vi "SP Perform Filter Attenuation Limit Testing.vi"(6 "Limit Results In":T3={"Limit #"=0, "Parameter"={"Stimulus Port"=1, "Response Port"=0}, "Bandwidth Pass?"={"Pass?"=FALSE, "Bandwidth"=0.0, "Limit"=0.0, "Units"=enum."Hz"}, "Ripple Pass?"={"Pass?"=FALSE, "Ripple"=0.0, "Limit"=0.0, "Format"=enum."Log Mag"}, "Attenuation Results"=[], "Skirt Results"=[], "Pass?"=FALSE} {"Parameter"."Stimulus Port" min=1 step=1; "Parameter"."Response Port" min=1 step=1}, 8 "error in (no error)":errorcluster, 10 "Data":T11={"F0"=500.0, "dF"=1.0, "Formatted Values"=[-6.0, -6.0, -6.0, -6.0, -6.0, -6.0, -5.0, -4.0, -3.0, -2.0, -1.0017226002993769, -0.8636286738753696, -1.012432061728755, -0.8135188671805874, -1.084383696215112, -1.192695586219516, -0.8228939725524264, -1.1588169801015764, -1.0069715761898415, -0.8118111488159718, -0.9516999033989667, -1.0842662636672022, -1.0261931083967077, -0.816874162233468, -0.8335770068326294, -1.1794529347576463, -1.1032959879886735, -1.197742447623333, -0.9631229100196212, -0.9908453124177325, -0.9835470980893588, -1.10217991844936, -0.8956607286257672, -0.8794782872077156, -0.9013683651609963, -1.0772188731817596, -0.992723355191172, -0.9536275499498994, -0.9874327685983141, -0.921963653527827, -0.8848787728556787, -1.1874980208218, -0.996957511881206, -0.9972503730309241, -0.8866139538542095, -1.07344181331393, -0.881559772443858, -1.0112449407130875, -0.9865384477979471, -0.9901446738263366, -1.1718630063784758, -0.9951725256878827, -0.931778781153855, -0.9846289731021831, -0.851763264124267, -0.9086965469391421, -0.8349429101974368, -0.8383742350256687, -1.106571816484691, -0.9554005266395742, -0.9376822403043366, -1.131287512516927, -1.0382288806403288, -0.917054052988136, -0.9489467877812984, -0.9264227759143271, -1.0918690925892351, -1.1668737446636852, -1.0021735712381068, -1.1541225361979714, -1.1931131329605709, -0.8730502330378824, -0.850411285659811, -1.137775166801135, -1.1870586525662095, -1.0926571181161528, -1.118993526927924, -1.1211410787283602, -0.8920697041785735, -0.888430731015914, -1.0656600076605476, -1.1666787859795846, -1.0713340188424678, -0.8625910088884297, -1.1434360227216422, -0.9217710376784376, -1.1218396445954617, -0.9558195687190933, -1.1773692443654946, -1.0827782751424972, -1.1567791336122029, -0.8684407402614696, -0.8177845157195978, -0.9040657051180614, -0.9313557288389804, -1.0236831450620423, -1.050426714979035, -0.8344777069605718, -0.8274082929927138, -1.1990080831766776, -1.0947798998491134, -1.1963114865246718, -1.0016247375583676, -1.0877110100652403, -1.1556028882288836, -1.1918380581525247, -0.9751292214691399, -0.8884133044813358, -1.0347444321214612, -0.9445125246491541, -2.0, -3.0, -4.0, -5.0, -6.0, -6.0, -6.0, -6.0, -6.0, -6.0]}, 11 "Filter Limit":T12={"Limit #"=1, "Parameter"={"Stimulus Port"=1, "Response Port"=2}, "Format"=enum."Lin Mag", "Filter Type"=enum."Bandpass", "Passband"={"Start/Center"=510.0, "Stop/Span"=610.0, "Units"=enum."MHz", "Freq Format"=enum."Start/Stop", "Bandwidth Attn"=3.0, "Passband Limit"=FALSE}, "Ripple"={"Ripple Limit"=TRUE, "Window On"=FALSE, "Ripple"=0.1, "Window"=10.0, "Units"=enum."MHz"}, "Attenuation Points"=[{"Attenuation"=3.0, "Type"=enum."Center", "Lower"=10.0, "Upper"=10.0, "Units"=enum."MHz"}], "Skirt Points"=[]} {"Parameter"."Stimulus Port" min=1 step=1; "Parameter"."Response Port" min=1 step=1; "Passband"."Bandwidth Attn" format="%.3g"; "Passband"."Stop/Span" format="%.3g"; "Passband"."Start/Center" format="%.3g"}) -> (0 "error out":errorcluster, 1 "Failures":cluster{"x values":dbl[], "y values":dbl[]}[](array[cluster]), 2 "Results":T2(array[cluster]), 3 "Pass?":bool=TRUE, 4 "Limit Results Out":T3={"Limit #"=0, "Parameter"={"Stimulus Port"=1, "Response Port"=0}, "Bandwidth Pass?"={"Pass?"=FALSE, "Bandwidth"=0.0, "Limit"=0.0, "Units"=enum."Hz"}, "Ripple Pass?"={"Pass?"=FALSE, "Ripple"=0.0, "Limit"=0.0, "Format"=enum."Log Mag"}, "Attenuation Results"=[], "Skirt Results"=[], "Pass?"=FALSE} {"Parameter"."Stimulus Port" min=1 step=1; "Parameter"."Response Port" min=1 step=1}, 5 "Lower Limits":cluster{"x values":dbl[], "y values":dbl[]}[](array[cluster])=[{"x values"=[550.0, 550.0], "y values"=[-inf, inf]}], 7 "Upper Limits":cluster{"x values":dbl[], "y values":dbl[]}[](array[cluster])=[{"x values"=[570.0, 570.0], "y values"=[-inf, inf]}])   [LabVIEW 2011]
uses:
  TypeDefs/SP Filter.ctl
  TypeDefs/SP Parameter.ctl
  TypeDefs/SP Format.ctl
  TypeDefs/SP Filter Type.ctl
  TypeDefs/SP Filter Passband.ctl
  TypeDefs/SP Frequency Units.ctl
  TypeDefs/SP Frequency Format.ctl
  TypeDefs/SP Filter Ripple.ctl
  TypeDefs/SP Attenuation Point.ctl
  TypeDefs/SP Attenuation Type.ctl
  TypeDefs/SP Skirt Rejection Point.ctl
  TypeDefs/SP Relative Loss.ctl
  TypeDefs/SP Limit Results.ctl
  TypeDefs/SP Bandwidth Limit Results.ctl
  TypeDefs/SP Ripple Limit Results.ctl
  TypeDefs/SP Attenuation Limit Results.ctl
  TypeDefs/SP Skirt Limit Results.ctl
panel:
  out "Plot Output":cluster{"x values":dbl[], "y values":dbl[]}[](graph)=[{"x values"=[], "y values"=[]}, {"x values"=[570.0, 570.0], "y values"=[-inf, inf]}, {"x values"=[550.0, 550.0], "y values"=[-inf, inf]}, {"x values"=[500.0, 501.0, 502.0, 503.0, 504.0, 505.0, 506.0, 507.0, 508.0, 509.0, 510.0, 511.0, 512.0, 513.0, 514.0, 515.0, 516.0, 517.0, 518.0, 519.0, 520.0, 521.0, 522.0, 523.0, 524.0, 525.0, 526.0, 527.0, 528.0, 529.0, 530.0, 531.0, 532.0, 533.0, 534.0, 535.0, 536.0, 537.0, 538.0, 539.0, 540.0, 541.0, 542.0, 543.0, 544.0, 545.0, 546.0, 547.0, 548.0, 549.0, 550.0, 551.0, 552.0, 553.0, 554.0, 555.0, 556.0, 557.0, 558.0, 559.0, 560.0, 561.0, 562.0, 563.0, 564.0, 565.0, 566.0, 567.0, 568.0, 569.0, 570.0, 571.0, 572.0, 573.0, 574.0, 575.0, 576.0, 577.0, 578.0, 579.0, 580.0, 581.0, 582.0, 583.0, 584.0, 585.0, 586.0, 587.0, 588.0, 589.0, 590.0, 591.0, 592.0, 593.0, 594.0, 595.0, 596.0, 597.0, 598.0, 599.0, 600.0, 601.0, 602.0, 603.0, 604.0, 605.0, 606.0, 607.0, 608.0, 609.0, 610.0, 611.0, 612.0, 613.0, 614.0, 615.0, 616.0, 617.0, 618.0, 619.0], "y values"=[-6.0, -6.0, -6.0, -6.0, -6.0, -6.0, -5.0, -4.0, -3.0, -2.0, -1.0017226002993769, -0.8636286738753696, -1.012432061728755, -0.8135188671805874, -1.084383696215112, -1.192695586219516, -0.8228939725524264, -1.1588169801015764, -1.0069715761898415, -0.8118111488159718, -0.9516999033989667, -1.0842662636672022, -1.0261931083967077, -0.816874162233468, -0.8335770068326294, -1.1794529347576463, -1.1032959879886735, -1.197742447623333, -0.9631229100196212, -0.9908453124177325, -0.9835470980893588, -1.10217991844936, -0.8956607286257672, -0.8794782872077156, -0.9013683651609963, -1.0772188731817596, -0.992723355191172, -0.9536275499498994, -0.9874327685983141, -0.921963653527827, -0.8848787728556787, -1.1874980208218, -0.996957511881206, -0.9972503730309241, -0.8866139538542095, -1.07344181331393, -0.881559772443858, -1.0112449407130875, -0.9865384477979471, -0.9901446738263366, -1.1718630063784758, -0.9951725256878827, -0.931778781153855, -0.9846289731021831, -0.851763264124267, -0.9086965469391421, -0.8349429101974368, -0.8383742350256687, -1.106571816484691, -0.9554005266395742, -0.9376822403043366, -1.131287512516927, -1.0382288806403288, -0.917054052988136, -0.9489467877812984, -0.9264227759143271, -1.0918690925892351, -1.1668737446636852, -1.0021735712381068, -1.1541225361979714, -1.1931131329605709, -0.8730502330378824, -0.850411285659811, -1.137775166801135, -1.1870586525662095, -1.0926571181161528, -1.118993526927924, -1.1211410787283602, -0.8920697041785735, -0.888430731015914, -1.0656600076605476, -1.1666787859795846, -1.0713340188424678, -0.8625910088884297, -1.1434360227216422, -0.9217710376784376, -1.1218396445954617, -0.9558195687190933, -1.1773692443654946, -1.0827782751424972, -1.1567791336122029, -0.8684407402614696, -0.8177845157195978, -0.9040657051180614, -0.9313557288389804, -1.0236831450620423, -1.050426714979035, -0.8344777069605718, -0.8274082929927138, -1.1990080831766776, -1.0947798998491134, -1.1963114865246718, -1.0016247375583676, -1.0877110100652403, -1.1556028882288836, -1.1918380581525247, -0.9751292214691399, -0.8884133044813358, -1.0347444321214612, -0.9445125246491541, -2.0, -3.0, -4.0, -5.0, -6.0, -6.0, -6.0, -6.0, -6.0, -6.0]}]
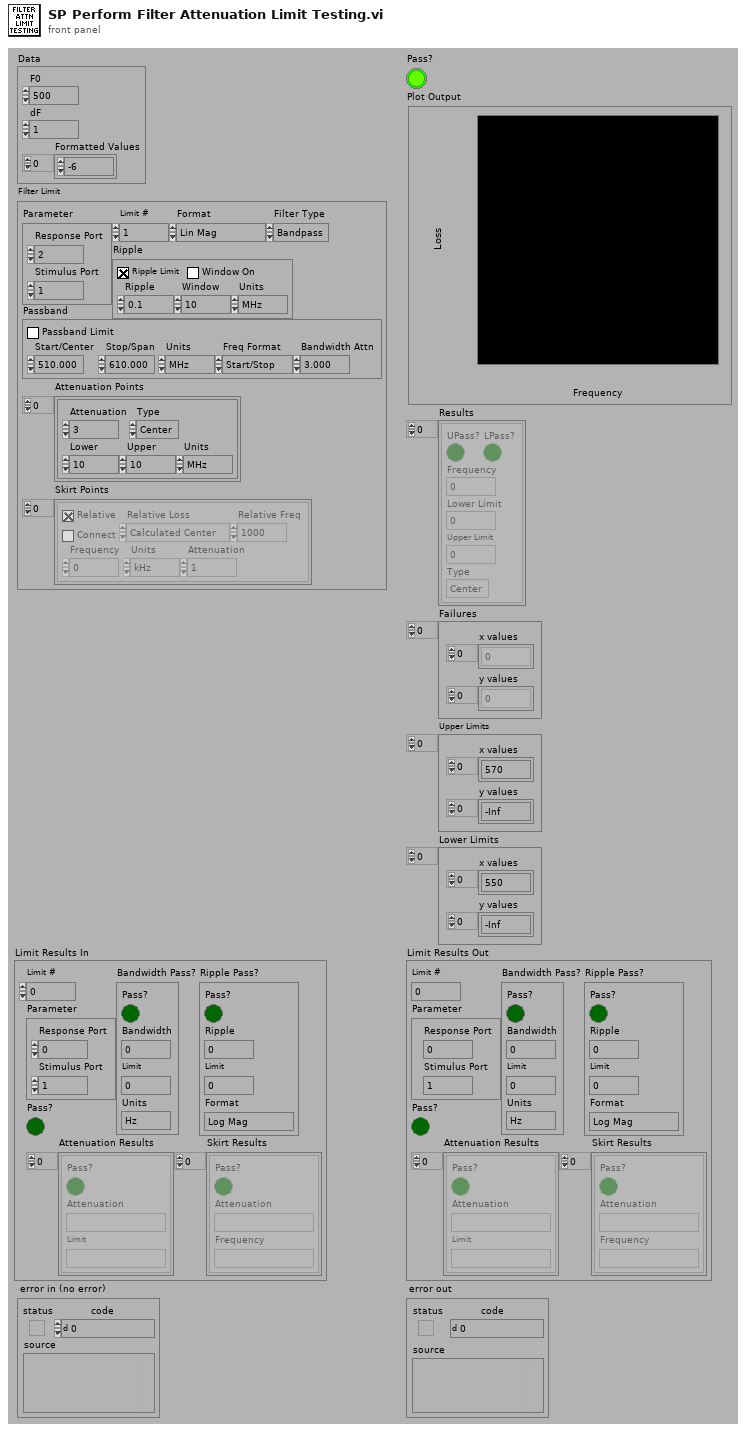
[diagram p1: front panel]
types:
  T1 = typedef "SP Attenuation Type.ctl" = enum16{"Center", "Lower", "Upper"}
  T2 = cluster{"UPass?":bool, "LPass?":bool, "Frequency":dbl, "Lower Limit":dbl, "Upper Limit":dbl, "Type":T1}[]
  T3 = typedef "SP Limit Results.ctl" = cluster{"Limit #":i8, "Parameter":T4, "Bandwidth Pass?":T5, "Ripple Pass?":T7, "Attenuation Results":T9[], "Skirt Results":T10[], "Pass?":bool}
  T4 = typedef "SP Parameter.ctl" = cluster{"Stimulus Port":i8, "Response Port":i8}
  T5 = typedef "SP Bandwidth Limit Results.ctl" = cluster{"Pass?":bool, "Bandwidth":dbl, "Limit":dbl, "Units":T6}
  T6 = typedef "SP Frequency Units.ctl" = enum16{"Hz", "kHz", "MHz", "GHz", "Points"}
  T7 = typedef "SP Ripple Limit Results.ctl" = cluster{"Pass?":bool, "Ripple":dbl, "Limit":dbl, "Format":T8}
  T8 = typedef "SP Format.ctl" = enum16{"Log Mag", "Lin Mag", "SWR", "Phase", "Expanded Phase", "Delay", "Insertion Loss", "Isolation", "Return Loss"}
  T9 = typedef "SP Attenuation Limit Results.ctl" = cluster{"Pass?":bool, "Attenuation":string, "Limit":string}
  T10 = typedef "SP Skirt Limit Results.ctl" = cluster{"Pass?":bool, "Attenuation":string, "Frequency":string}
  T11 = cluster{"F0":dbl, "dF":dbl, "Formatted Values":dbl[]}
  T12 = typedef "SP Filter.ctl" = cluster{"Limit #":i8, "Parameter":T4, "Format":T8, "Filter Type":T13, "Passband":T14, "Ripple":T16, "Attenuation Points":T17[], "Skirt Points":T18[]}
  T13 = typedef "SP Filter Type.ctl" = enum16{"Lowpass", "Highpass", "Bandpass", "Bandstop"}
  T14 = typedef "SP Filter Passband.ctl" = cluster{"Start/Center":dbl, "Stop/Span":dbl, "Units":T6, "Freq Format":T15, "Bandwidth Attn":dbl, "Passband Limit":bool}
  T15 = typedef "SP Frequency Format.ctl" = enum16{"Start/Stop", "Center/Span"}
  T16 = typedef "SP Filter Ripple.ctl" = cluster{"Ripple Limit":bool, "Window On":bool, "Ripple":dbl, "Window":dbl, "Units":T6}
  T17 = typedef "SP Attenuation Point.ctl" = cluster{"Attenuation":dbl, "Type":T1, "Lower":dbl, "Upper":dbl, "Units":T6}
  T18 = typedef "SP Skirt Rejection Point.ctl" = cluster{"Relative":bool, "Connect":bool, "Frequency":dbl, "Units":T6, "Attenuation":dbl, "Relative Loss":T19, "Relative Freq":dbl}
  T19 = typedef "SP Relative Loss.ctl" = enum16{"Calculated Center", "Passband Minimum", "Passband Maximum", "Passband Average", "Frequency"}
  T20 = cluster{bool, bool, "Interpolated X Value":dbl, dbl, dbl, "Type":T1}
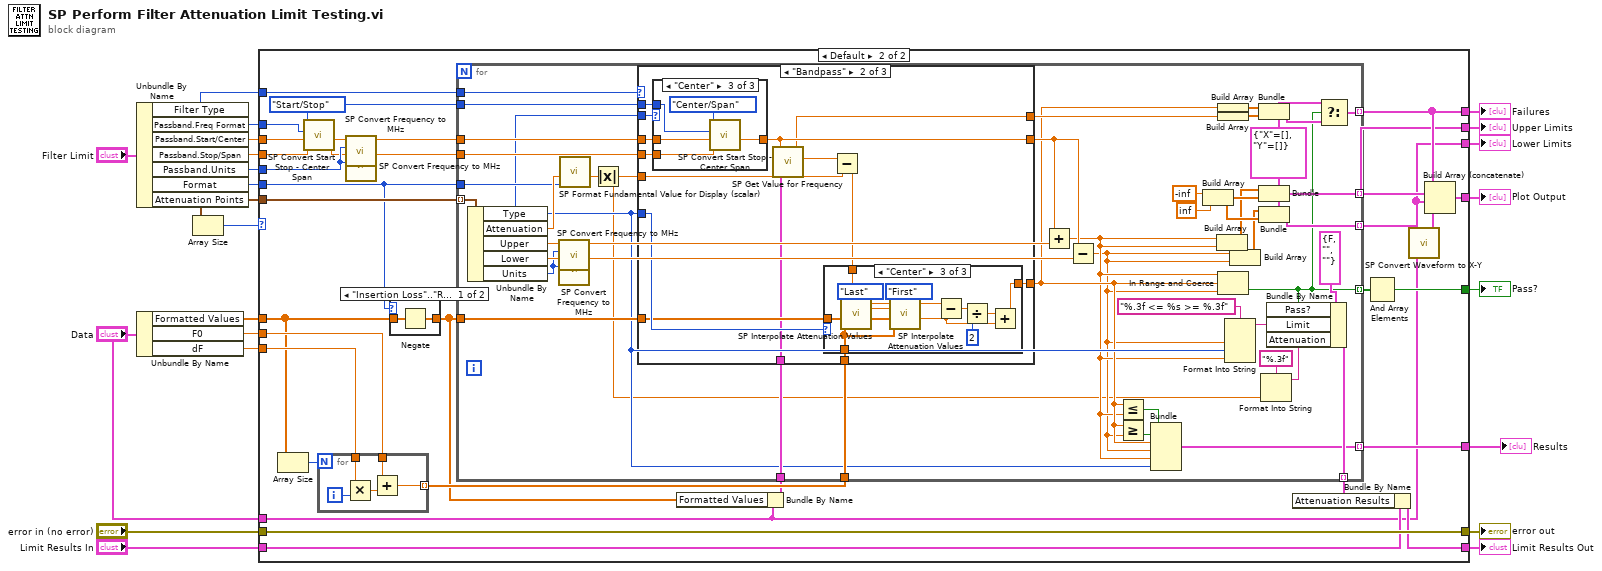
[diagram p0: block diagram]
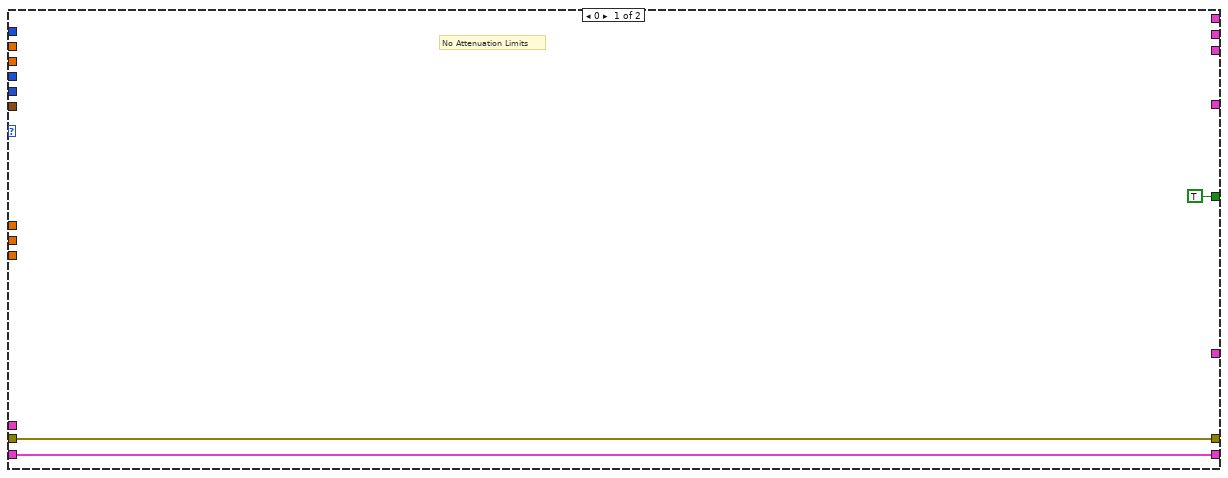
[diagram p2: hidden frame]
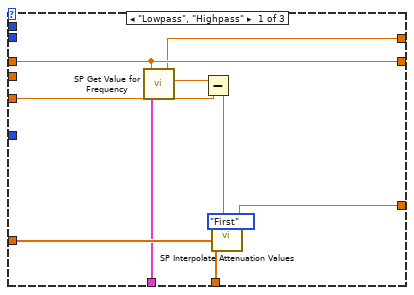
[diagram p4: hidden frame]
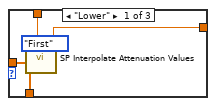
[diagram p5: hidden frame]
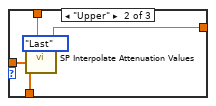
[diagram p6: hidden frame]
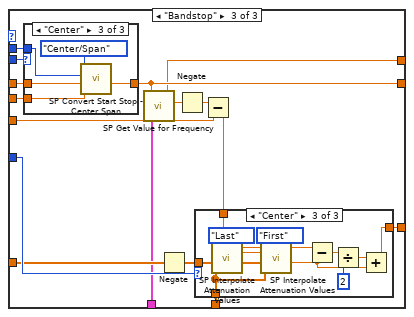
[diagram p9: hidden frame]
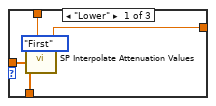
[diagram p10: hidden frame]
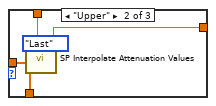
[diagram p11: hidden frame]
diagram:
  n1 = Unbundle By Name("Filter Limit") -> ("Filter Type"=w14:T13, "Passband.Freq Format"=w13:T15, "Passband.Start/Center"=w22:dbl, "Passband.Stop/Span"=w21:dbl, "Passband.Units"=w20:T6, "Format"=w11:T8, "Attenuation Points"=w12:T17[])
  n2 = Unbundle By Name("Data") -> ("Formatted Values"=w19:dbl[], "F0"=w8:dbl, "dF"=w7:dbl)
  n3 = Array Size(array=w12) -> (size(s)=w9:i32)
  n4 = case shown="Default" w9 {
    tunnel: w14 -> [_ w49]
    tunnel: w22 -> [_ w55]
    tunnel: w21 -> [_ w52]
    tunnel: w20 -> [_ w58]
    tunnel: w19 -> [_ w31]
    tunnel: w12 -> [_ w56]
    tunnel: "Data" -> [_ w29]
    tunnel: [TRUE w46] -> w17
    tunnel: "error in (no error)" -> [w26 w45]
    tunnel: [w26 w45] -> w15
    tunnel: w13 -> [_ w51]
    tunnel: w11 -> [_ w30]
    tunnel: [_ w48] -> w10
    tunnel: w8 -> [_ w41]
    tunnel: w7 -> [_ w40]
    tunnel: [_ w39] -> w6
    tunnel: [_ w38] -> w5
    tunnel: [_ w37] -> w4
    tunnel: "Limit Results In" -> [w24 w34]
    tunnel: [w24 w33] -> w2
    tunnel: [_ w32] -> w1
    frame 0 {
      # "No Attenuation Limits"
    }
    frame Default {
      w42 = SP_Frequency_Format."Start/Stop" ("Freq Format To")
      n5 = Array Size(array=w31) -> (size(s)=w44:i32)
      n6 = call "SP Convert Start Stop - Center Span.vi"("Stop/Span In"=w52, "Start/Center In"=w55, "Freq Format From"=w51, "Freq Format To"=w42) -> ("Stop/Span Out"=w53:dbl, "Start/Center Out"=w54:dbl)  [unwired: 6 out]
      n7 = for {
        N: w44 -> [_]
        tunnel: w40 -> [w65]
        tunnel: w41 -> [w63]
        tunnel: [w62] -> w43 mode=indexing
        i -> [w66]
        n8 = Multiply(x=w65, y=w66) -> (x*y=w64:dbl)
        n9 = Add(x=w63, y=w64) -> (x+y=w62:dbl)
      }
      n10 = call "SP Convert Frequency to MHz.vi"("Units"=w58, "Frequency"=w54) -> ("Converted Frequency"=w50:dbl)  [unwired: 1 in, 8 out]
      n11 = call "SP Convert Frequency to MHz.vi"("Units"=w58, "Frequency"=w53) -> ("Converted Frequency"=w57:dbl)  [unwired: 1 in, 8 out]
      n12 = case shown="\"Insertion Loss\"..\"Return Loss\"" w30 {
        tunnel: w31 -> [w60 w61]
        tunnel: [w59 w61] -> w27
        frame "Insertion Loss".."Return Loss" {
          n13 = Negate(x=w60) -> (-x=w59:dbl[])
        }
        frame Default {
        }
      }
      n14 = Bundle By Name(cluster=w29, "Formatted Values"=w27) -> (w28:T11)
      n15 = for {
        tunnel: w49 -> [w111]
        tunnel: w27 -> [w104]
        tunnel: w57 -> [w110]
        tunnel: w50 -> [w95]
        tunnel: w56 -> [w109] mode=indexing
        tunnel: [w94] -> w38 mode=indexing
        tunnel: [w93] -> w37 mode=indexing
        tunnel: w30 -> [w90]
        tunnel: [w73] -> w36 mode=indexing
        tunnel: w43 -> [w105]
        tunnel: w42 -> [w103]
        tunnel: w28 -> [w89]
        tunnel: [w85] -> w39 mode=indexing
        tunnel: [w82] -> w35 mode=indexing
        tunnel: [w74] -> w32 mode=indexing
        w84 = cluster{"X":dbl[], "Y":dbl[]} {"X"=[], "Y"=[]} ("Cluster")
        n16 = Unbundle By Name(w109) -> ("Type"=w75:T1, "Attenuation"=w91:dbl, "Upper"=w108:dbl, "Lower"=w107:dbl, "Units"=w106:T6)
        n17 = call "SP Convert Frequency to MHz.vi"("Units"=w106, "Frequency"=w108) -> ("Converted Frequency"=w97:dbl)  [unwired: 1 in, 8 out]
        n18 = call "SP Convert Frequency to MHz.vi"("Units"=w106, "Frequency"=w107) -> ("Converted Frequency"=w96:dbl)  [unwired: 1 in, 8 out]
        n19 = call "SP Format Fundamental Value for Display (scalar).vi"("Format"=w90, "Stored Value (0, linear)"=w91) -> ("Display Value"=w79:dbl)  [unwired: 5 out]
        n20 = Absolute Value(x=w79) -> (abs(x)=w67:dbl)
        n21 = case shown="\"Bandpass\"" w111 {
          tunnel: w110 -> [_ w130 w173]
          tunnel: w95 -> [w114 w131 w174]
          tunnel: w104 -> [w116 w125 w167]
          tunnel: w105 -> [w120 w133 w176]
          tunnel: w67 -> [w117 w126 w166]
          tunnel: w75 -> [_ w132 w175]
          tunnel: w103 -> [_ w129 w172]
          tunnel: w75 -> [_ w128 w171]
          tunnel: [w118 w127 w168] -> w72
          tunnel: [w114 w124 w165] -> w92
          tunnel: w89 -> [w115 w123 w164]
          tunnel: [w113 w121 w163] -> w86
          frame "Lowpass", "Highpass" {
            n22 = call "SP Get Value for Frequency.vi"("Data"=w115, "Frequency (MHz)"=w114) -> ("Value"=w113:dbl)  [unwired: 5 out]
            n23 = Subtract(x=w113, y=w117) -> (x-y=w112:dbl)
            n24 = call "SP Interpolate Attenuation Values.vi"("Instance (First)"=enum16{"First", "Last"}."First", "Attenuation Value"=w112, "X Values"=w120, "Y Values"=w116) -> ("Interpolated X Value"=w118:dbl)  [unwired: 7 out]
          }
          frame "Bandpass" {
            n25 = case shown="\"Center\"" w132 {
              tunnel: w131 -> [w155 _ w160]
              tunnel: w130 -> [_ w156 w159]
              tunnel: [w155 w156 w157] -> w124
              tunnel: w129 -> [_ _ w158]
              frame "Lower" {
              }
              frame "Upper" {
              }
              frame "Center" {
                n26 = call "SP Convert Start Stop - Center Span.vi"("Stop/Span In"=w159, "Start/Center In"=w160, "Freq Format From"=w158, "Freq Format To"=SP_Frequency_Format."Center/Span") -> ("Start/Center Out"=w157:dbl)  [unwired: 7 out]
              }
            }
            n27 = call "SP Get Value for Frequency.vi"("Data"=w123, "Frequency (MHz)"=w124) -> ("Value"=w121:dbl)  [unwired: 5 out]
            n28 = Subtract(x=w121, y=w126) -> (x-y=w122:dbl)
            n29 = case shown="\"Center\"" w128 {
              tunnel: w133 -> [w138 w143 w151]
              tunnel: [w137 w142 w145] -> w127
              tunnel: w125 -> [w136 w141 w152]
              tunnel: w122 -> [w135 w140 w150]
              frame "Lower" {
                n30 = call "SP Interpolate Attenuation Values.vi"("Instance (First)"=enum16{"First", "Last"}."First", "Attenuation Value"=w135, "X Values"=w138, "Y Values"=w136) -> ("Interpolated X Value"=w137:dbl)  [unwired: 7 out]
              }
              frame "Upper" {
                n31 = call "SP Interpolate Attenuation Values.vi"("Instance (First)"=enum16{"First", "Last"}."Last", "Attenuation Value"=w140, "X Values"=w143, "Y Values"=w141) -> ("Interpolated X Value"=w142:dbl)  [unwired: 7 out]
              }
              frame "Center" {
                n32 = call "SP Interpolate Attenuation Values.vi"("Instance (First)"=enum16{"First", "Last"}."Last", "Attenuation Value"=w150, "X Values"=w151, "Y Values"=w152) -> ("Interpolated X Value"=w149:dbl)  [unwired: 7 out]
                n33 = call "SP Interpolate Attenuation Values.vi"("Instance (First)"=enum16{"First", "Last"}."First", "Attenuation Value"=w150, "X Values"=w151, "Y Values"=w152) -> ("Interpolated X Value"=w144:dbl)  [unwired: 7 out]
                n34 = Subtract(x=w149, y=w144) -> (x-y=w148:dbl)
                n35 = Divide(x=w148, y=i8 2) -> (x/y=w146:dbl)
                n36 = Add(x=w146, y=w144) -> (x+y=w145:dbl)
              }
            }
          }
          frame "Bandstop" {
            n37 = case shown="\"Center\"" w175 {
              tunnel: w174 -> [w198 _ w203]
              tunnel: w173 -> [_ w199 w202]
              tunnel: [w198 w199 w200] -> w165
              tunnel: w172 -> [_ _ w201]
              frame "Lower" {
              }
              frame "Upper" {
              }
              frame "Center" {
                n38 = call "SP Convert Start Stop - Center Span.vi"("Stop/Span In"=w202, "Start/Center In"=w203, "Freq Format From"=w201, "Freq Format To"=SP_Frequency_Format."Center/Span") -> ("Start/Center Out"=w200:dbl)  [unwired: 7 out]
              }
            }
            n39 = call "SP Get Value for Frequency.vi"("Data"=w164, "Frequency (MHz)"=w165) -> ("Value"=w163:dbl)  [unwired: 5 out]
            n40 = Negate(x=w167) -> (-x=w170:dbl[])
            n41 = Negate(x=w163) -> (-x=w169:dbl)
            n42 = Subtract(x=w169, y=w166) -> (x-y=w162:dbl)
            n43 = case shown="\"Center\"" w171 {
              tunnel: w176 -> [w181 w186 w194]
              tunnel: [w180 w185 w188] -> w168
              tunnel: w170 -> [w179 w184 w195]
              tunnel: w162 -> [w178 w183 w193]
              frame "Lower" {
                n44 = call "SP Interpolate Attenuation Values.vi"("Instance (First)"=enum16{"First", "Last"}."First", "Attenuation Value"=w178, "X Values"=w181, "Y Values"=w179) -> ("Interpolated X Value"=w180:dbl)  [unwired: 7 out]
              }
              frame "Upper" {
                n45 = call "SP Interpolate Attenuation Values.vi"("Instance (First)"=enum16{"First", "Last"}."Last", "Attenuation Value"=w183, "X Values"=w186, "Y Values"=w184) -> ("Interpolated X Value"=w185:dbl)  [unwired: 7 out]
              }
              frame "Center" {
                n46 = call "SP Interpolate Attenuation Values.vi"("Instance (First)"=enum16{"First", "Last"}."Last", "Attenuation Value"=w193, "X Values"=w194, "Y Values"=w195) -> ("Interpolated X Value"=w192:dbl)  [unwired: 7 out]
                n47 = call "SP Interpolate Attenuation Values.vi"("Instance (First)"=enum16{"First", "Last"}."First", "Attenuation Value"=w193, "X Values"=w194, "Y Values"=w195) -> ("Interpolated X Value"=w187:dbl)  [unwired: 7 out]
                n48 = Subtract(x=w192, y=w187) -> (x-y=w191:dbl)
                n49 = Divide(x=w191, y=i8 2) -> (x/y=w189:dbl)
                n50 = Add(x=w189, y=w187) -> (x+y=w188:dbl)
              }
            }
          }
        }
        n51 = Add(x=w92, y=w97) -> (x+y=w71:dbl)
        n52 = Subtract(x=w92, y=w96) -> (x-y=w70:dbl)
        n53 = Less Or Equal?(x=w72, y=w71) -> (x <= y?=w69:bool)
        n54 = Greater Or Equal?(x=w72, y=w70) -> (x >= y?=w68:bool)
        n55 = Bundle(w69, w68, "Interpolated X Value"=w72, w70, w71, "Type"=w75) -> (w74:T20)  [unwired: 1 out]
        n56 = Build Array(-inf ("Numeric"), inf ("Numeric")) -> (w100:dbl[])
        n57 = Build Array(w71, w71) -> (w98:dbl[])
        n58 = Build Array(w72) -> (w88:dbl[])
        n59 = Build Array(w86) -> (w87:dbl[])
        n60 = In Range and Coerce(upper limit=w71, x=w72, lower limit=w70) -> (In Range?=w73:bool)  [unwired: 1 out]
        n61 = Format Into String(format string="%.3f <= %s >= %.3f", w70, w75, w71) -> (resulting string=w77:string)  [unwired: 2 in, 1 out]
        n62 = Build Array(w70, w70) -> (w99:dbl[])
        n63 = Bundle(cluster=w84, "X"=w88, "Y"=w87) -> (w83:cluster{"X":dbl[], "Y":dbl[]})
        n64 = Bundle(cluster=w84, "X"=w98, "Y"=w100) -> (w94:cluster{"X":dbl[], "Y":dbl[]})
        n65 = Bundle(cluster=w84, "X"=w99, "Y"=w100) -> (w93:cluster{"X":dbl[], "Y":dbl[]})
        n66 = Format Into String(format string="%.3f", w67) -> (resulting string=w80:string)  [unwired: 2 in, 1 out]
        n67 = Bundle By Name(cluster=T9 {"Pass?"=FALSE, "Attenuation"="", "Limit"=""} ("element"), "Pass?"=w73, "Limit"=w77, "Attenuation"=w80) -> (w82:T9)
        n68 = Select(t=w84, s=w73, f=w83) -> (s? t:f=w85:cluster{"X":dbl[], "Y":dbl[]})
      }
      n69 = Bundle By Name(cluster=w34, "Attenuation Results"=w35) -> (w33:T3)
      n70 = And Array Elements(Boolean array=w36) -> (logical AND=w46:bool)
      n71 = call "SP Convert Waveform to X-Y.vi"("Waveform"=w29) -> ("X-Y"=w47:cluster{"X":dbl[], "Y":dbl[]})
      n72 = Build Array (concatenate)(w39, w38, w37, w47) -> (w48:cluster{"X":dbl[], "Y":dbl[]}[])
    }
  }
  "Pass?" <- w17
  "Plot Output" <- w10
  "error out" <- w15
  "Upper Limits" <- w5
  "Lower Limits" <- w4
  "Failures" <- w6
  "Limit Results Out" <- w2
  "Results" <- w1
